vi "Type-T-Thermocouple_Init.vi"(8 "error in (no error)":errorcluster, 11 "object in":refnum<class "Type-T-Thermocouple.lvclass">) -> (0 "error out":errorcluster, 3 "object out":refnum<class "Type-T-Thermocouple.lvclass">)   [LabVIEW 2016, in "Type-T-Thermocouple.lvclass"]
uses:
  Type-T-Thermocouple.lvclass
  Type-T-Thermocouple.lvclass/Type-T-Thermocouple.ctl
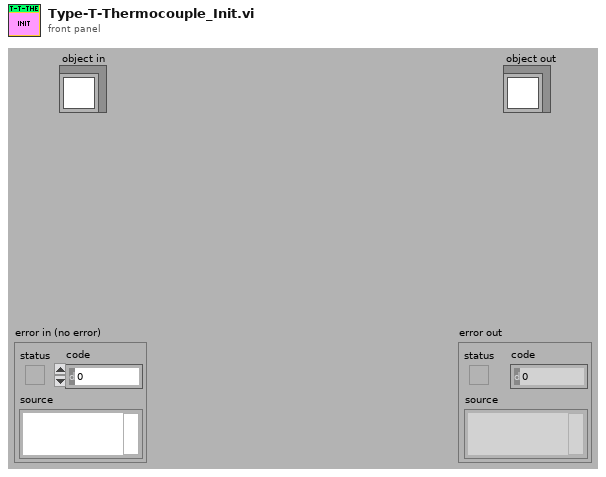
[diagram p1: front panel]
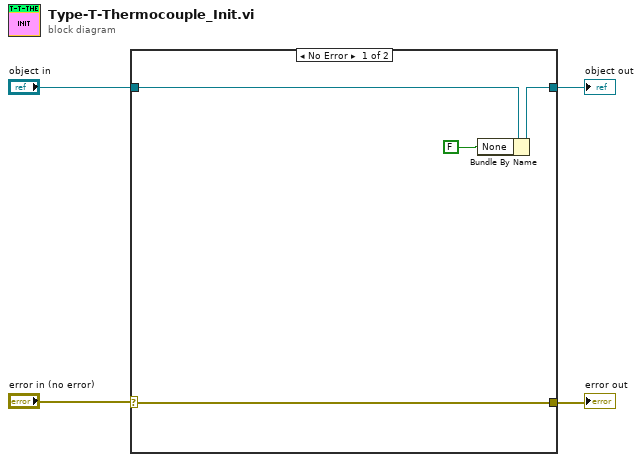
[diagram p0: block diagram]
diagram:
  n1 = case shown="No Error" "error in (no error)" {
    selector: "error in (no error)" -> [w5 w9]
    tunnel: "object in" -> [w8 w10]
    tunnel: [w7 w10] -> w3
    tunnel: [w5 w9] -> w1
    frame No Error {
      n2 = Bundle By Name(cluster=w8, "None"=FALSE) -> (w7:refnum<class "Type-T-Thermocouple.lvclass">)
    }
    frame Error {
    }
  }
  "object out" <- w3
  "error out" <- w1
